vi "14_DC Motor_cts2cm.vi"() -> ()   [LabVIEW 2018]
uses:
  <userlib>/KNR OS 4.0 LabVIEW Toolkit/Type Definition/Resource.ctl
  <userlib>/KNR OS 4.0 LabVIEW Toolkit/Type Definition/DC Motor Port.ctl
panel:
  in  "Speed (+-100%)":dbl(slide) scale=-100.0..100.0
  in  "IP":string(combo)="172.22.11.2"
  in  "Port":T1=4 items=["DS1"=4, "DS2"=5, "DS3"=6, "DS4"=7]
  in  "Resource":T2=enum."KNRm_DDDD"
  in  "stop":bool
  in  "Enable Motor":bool
  out "Position cm":dbl
  out "Velocity (cm/sec)":dbl
  in  "Reverse?":bool
  in  "Reset":bool
  # "KNR/KNRm\nPort5=DS1\nPort6=DS2\nPort7=DS3\nPort8=DS4"
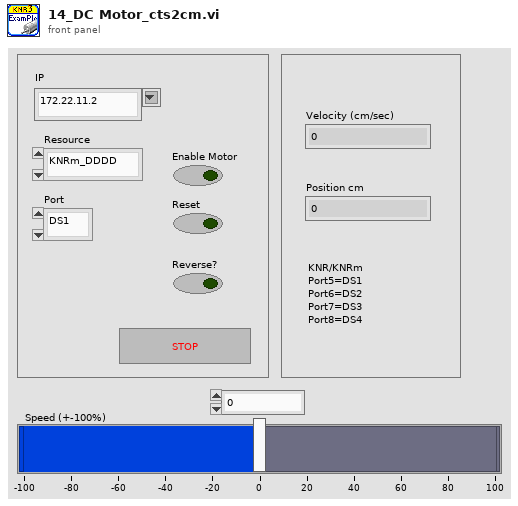
[diagram p1: front panel]
types:
  T1 = typedef "DC Motor Port.ctl" = u16
  T2 = typedef "Resource.ctl" = enum16{"KNRm_DDRC", "KNRm_DDDD", "KNRm_DDDR", "KNRm_DDDC", "KNR", "KNRm_neww"}
  T3 = typedef "KNR3 Reference.ctl" = cluster{"FPGA Session":refnum<class "FPGA Interface Base.lvclass">, "Resource":T2}
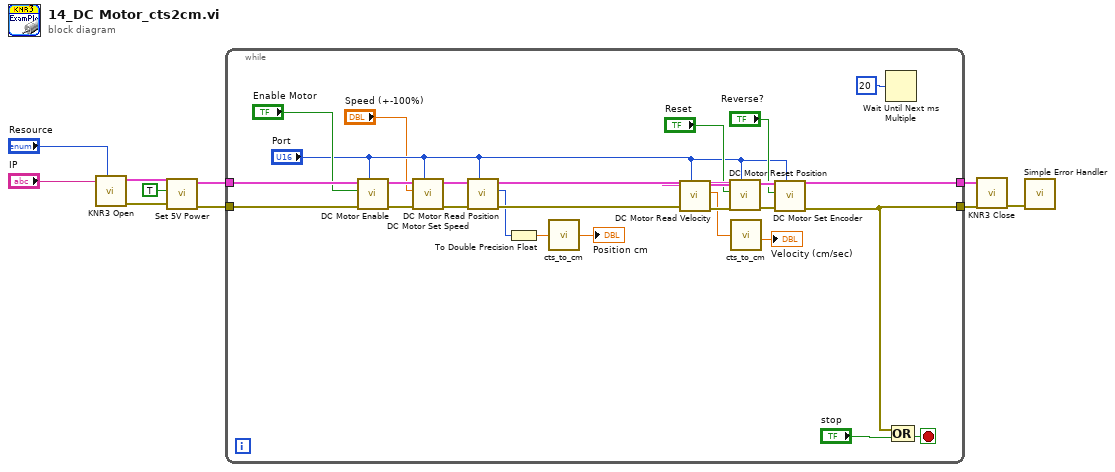
[diagram p0: block diagram]
diagram:
  n1 = call <userlib>:"KNR3 Open.vi"("Resource"="Resource", "IP"="IP") -> ("error out"=w2:errorcluster, "KNR out"=w4:T3)  [unwired: 8 in]
  n2 = call <userlib>:"Set 5V Power.vi"("error in (no error)"=w2, "5V Power(T)"=TRUE ("5V Power"), "KNR in"=w4) -> ("error out"=w8:errorcluster, "KNR out"=w9:T3)  [unwired: 7 in]
  n3 = while {
    tunnel: w9 -> [w37]
    tunnel: w8 -> [w33]
    tunnel: [w22] -> w6
    tunnel: [w23] -> w7
    stop <- w29 stop-if-true
    n4 = call <userlib>:"DC Motor Enable.vi"("Port (DS1)"="Port", "error in (no error)"=w33, "Enable Motor(F)"="Enable Motor", "KNR in"=w37) -> ("error out"=w32:errorcluster, "KNR out"=w36:T3)  [unwired: 6 in]
    n5 = call <userlib>:"DC Motor Set Speed.vi"("Port (DS1)"="Port", "error in (no error)"=w32, "Speed (+-100%)"="Speed (+-100%)", "KNR in"=w36) -> ("error out"=w31:errorcluster, "KNR out"=w35:T3)  [unwired: 6 in]
    n6 = call <userlib>:"DC Motor Read Position.vi"("Port (DS1)"="Port", "error in (no error)"=w31, "KNR in"=w35) -> ("error out"=w26:errorcluster, "Position"=w14:i32, "KNR out"=w27:T3)  [unwired: 6 in]
    n7 = To Double Precision Float(number=w14) -> (double precision float=w12:dbl)
    n8 = call "cts_to_cm.vi"("cts"=w12) -> ("cm"=→"Position cm":dbl)
    n9 = call <userlib>:"DC Motor Read Velocity.vi"("Port (DS1)"="Port", "error in (no error)"=w26, "KNR in"=w27) -> ("error out"=w20:errorcluster, "Velocity (cts/sec)"=w19:dbl, "KNR out"=w25:T3)  [unwired: 6 in]
    n10 = call <userlib>:"DC Motor Reset Position.vi"("Port (DS1)"="Port", "error in (no error)"=w20, "Reset(F)"="Reset", "KNR in"=w25) -> ("error out"=w21:errorcluster, "KNR out"=w24:T3)  [unwired: 6 in]
    n11 = call "cts_to_cm.vi"("cts"=w19) -> ("cm"=→"Velocity (cm/sec)":dbl)
    n12 = call <userlib>:"DC Motor Set Encoder.vi"("Port (DS1)"="Port", "error in (no error)"=w21, "Reverse?(F)"="Reverse?", "KNR in"=w24) -> ("error out"=w22:errorcluster, "KNR out"=w23:T3)  [unwired: 6 in]
    n13 = Wait Until Next ms Multiple(millisecond multiple=u32 20) -> ()  [unwired: 1 out]
    n14 = Compound Arithmetic op=OR(w22, "stop") -> (w29:bool)
  }
  n15 = call <userlib>:"KNR3 Close.vi"("error in (no error)"=w6, "KNR in"=w7) -> ("error out"=w5:errorcluster)  [unwired: 9 in]
  n16 = call <vilib>:"Simple Error Handler.vi"("error in (no error)"=w5) -> ()  [unwired: 4 in, 5 out]
